vi "3D_Ribbon_Plot_Merge_VI.vi"() -> ()   [LabVIEW 2020]
uses:
  <vilib>/Math Plots/3D Math Plots/3D Ribbon/3D Ribbon XCtrl/3D Ribbon.xctl
  <vilib>/Math Plots/3D Math Plots/3D Ribbon/3D Ribbon Datatype/Public/Plot Helper (Standard).vi
  <vilib>/Math Plots/3D Math Plots/3D Ribbon/3D Ribbon Datatype/3D Ribbon Datatype.lvclass
panel:
  out "3D Ribbon":refnum<class "3D Plot Datatype.lvclass">[](xcontrol)
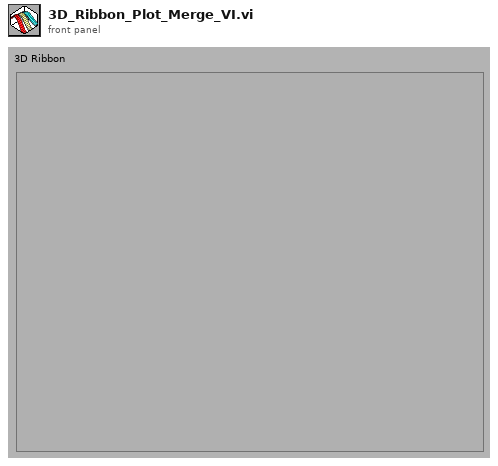
[diagram p1: front panel]
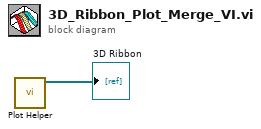
[diagram p0: block diagram]
diagram:
  n1 = call-poly <vilib>:"Plot Helper.vi"() -> ("3D Plot lvclass Array out"=→"3D Ribbon":refnum<class "3D Plot Datatype.lvclass">[])  [unwired: 5 in, 6 out]
